vi "Launcher.vi"() -> ()   [LabVIEW 2020]
uses:
  <userlib>/_NEVSTOP/Communicable State Machine(CSM)/_Support/GlobalEvent/GEvt-Convert Filter Rules - v1.0.vi
  <userlib>/_NEVSTOP/Communicable State Machine(CSM)/addons/INI-Static-Variable-Support/_Support/instances/_CSM - Read Log Filter Rules - v1.0.vi
  <userlib>/_NEVSTOP/Communicable State Machine(CSM)/_Support/GlobalEvent/LogFilter/SettingVIs/Set Global CSM Filter.vi
  <userlib>/_NEVSTOP/Communicable State Machine(CSM)/_Support/GlobalEvent/LogFilter/SettingVIs/Set Global LogType Filter.vi
  <userlib>/_NEVSTOP/Communicable State Machine(CSM)/_Support/GlobalEvent/LogFilter/SettingVIs/Set Global State Filter.vi
  <userlib>/_NEVSTOP/Communicable State Machine(CSM)/_Support/GlobalEvent/LogFilter/SettingVIs/Set CSM LogType Filter.vi
  <userlib>/_NEVSTOP/Communicable State Machine(CSM)/_Support/GlobalEvent/LogFilter/SettingVIs/Set CSM State Filter.vi
  <userlib>/_NEVSTOP/Communicable State Machine(CSM)/_Support/GlobalEvent/LogFilter/SettingVIs/Set Global StateType Filter.vi
  <userlib>/_NEVSTOP/Communicable State Machine(CSM)/_Support/GlobalEvent/LogFilter/SettingVIs/Set CSM StateType Filter.vi
  <userlib>/_NEVSTOP/Communicable State Machine(CSM)/addons/INI-Static-Variable-Support/_Support/instances/_CSM - Read File Logger Configuration - v1.0.vi
  src/resource/global-rc-strings.vi
  <userlib>/_NEVSTOP/Communicable State Machine(CSM)/_Support/GlobalEvent/LogFilter/LogFilter.lvclass
  <userlib>/_NEVSTOP/Communicable State Machine(CSM)/addons/Watchdog/CSM Watchdog.lvlib
  <userlib>/_NEVSTOP/Communicable State Machine(CSM)/addons/Logger/CSM File Logger.lvlib
  <userlib>/_NEVSTOP/Communicable State Machine(CSM)/Communicable State Machine.lvlib
  <userlib>/_NEVSTOP/Communicable State Machine(CSM)/addons/INI-Static-Variable-Support/INI-Static-Variable-Support.lvlib
  src/CSMScript-Engine(Lite).lvlib
panel:
  out "Information":string="Load \"csm\"..."
  out "CSMVersion":string="Powered By CSM, Copyright ?2025 NEVSTOP-LAB"
  out "CSMScript(version)":string="CSMScript-Lite"
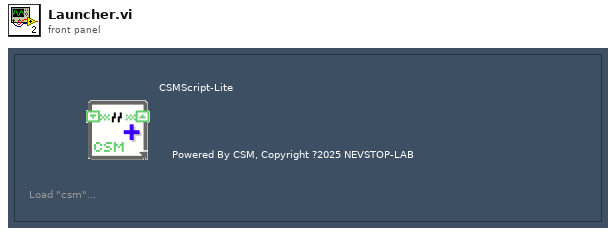
[diagram p1: front panel]
types:
  T1 = cluster{"Enable":bool, "Limit":cluster{"FileSize":i64, "FileNum":i32}, "Timestamp.Format":string, "AutoExit":bool}
  T2 = typedef "Communicable State Machine.lvlib/_CSM_GlobalLog Filter Rules - v1.0.ctl" = cluster{"Global":cluster{"CSM":string[], "LogType":T3[], "State":string[], "StateType":T4[]}, "CSM":cluster{"LogType":cluster{"CSM":string, "LogType":T3}[], "State":cluster{"CSM":string, "State":string}[], "StateType":cluster{"CSM":string, "LogType":T4}[]}}
  T3 = typedef "Communicable State Machine.lvlib/_CSM_GlobalLog_MSG_TYPE.ctl" = enum16{"User Log", "State Change", "Status", "Interrupt", "Register", "Unregister", "Error Log", "Module Created", "Module Destroyed", "Async Message", "No-Rep Async Message", "Sync Message", "AsyncMsg Complete", "SyncMsg Complete"}
  T4 = typedef "Communicable State Machine.lvlib/_CSM_GlobalLog_STATE_TYPE.ctl" = enum16{"State - Internal State", "State - External Message", "State - Response", "State - Complete"}
  T5 = enum32{"Invalid", "Standard", "Closed", "Hidden", "Minimized", "Maximized"}
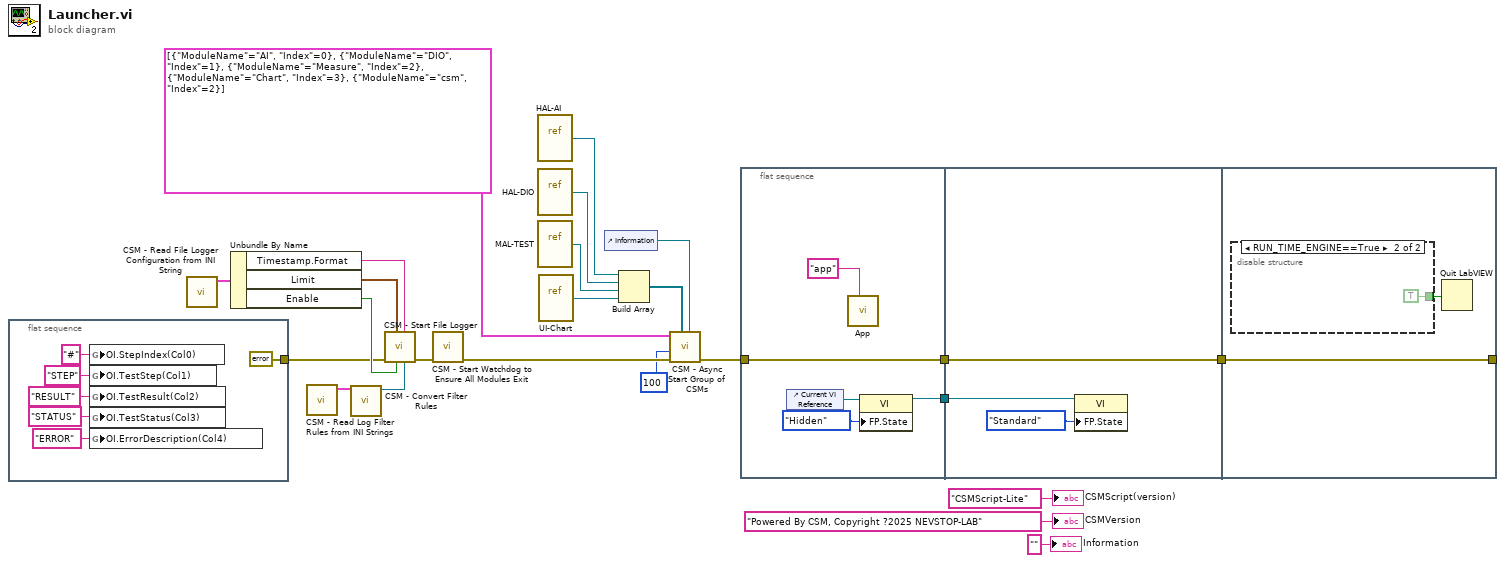
[diagram p0: block diagram]
diagram:
  n1 = flat-sequence {
    tunnel: [errorcluster {"status"=FALSE, "code"=0, "source"=""} ("error in (no error)")] -> w1
    frame #0 {
      n2 = global write "global-rc-strings.vi" "OI.StepIndex(Col0)"("#" ("OI.StepIndex(Col0)")) -> ()
      n3 = global write "global-rc-strings.vi" "OI.TestStep(Col1)"("STEP" ("OI.TestStep(Col1)")) -> ()
      n4 = global write "global-rc-strings.vi" "OI.TestResult(Col2)"("RESULT" ("OI.TestResult(Col2)")) -> ()
      n5 = global write "global-rc-strings.vi" "OI.TestStatus(Col3)"("STATUS" ("OI.TestStatus(Col3)")) -> ()
      n6 = global write "global-rc-strings.vi" "OI.ErrorDescription(Col4)"("ERROR" ("OI.TestStatus(Col3)")) -> ()
    }
  }
  n7 = call-poly <userlib>:"CSM - Read File Logger Configuration from INI String.vi"() -> ("FileLogger Configuration-v1"=w11:T1)  [unwired: 8 in, 1 out]
  n8 = Unbundle By Name(w11) -> ("Timestamp.Format"=w8:string, "Limit"=w9:cluster{"FileSize":i64, "FileNum":i32}, "Enable"=w10:bool)
  n9 = call-poly <userlib>:"CSM - Read Log Filter Rules from INI Strings.vi"() -> ("Rules-v1"=w13:T2)  [unwired: 8 in, 1 out]
  n10 = call-poly <userlib>:"CSM - Convert Filter Rules.vi"("Rules-v1"=w13) -> ("GlobalLogFilter"=w14:refnum<class "LogFilter.lvclass">)  [unwired: 10 in]
  n11 = call <userlib>:"CSM - Start File Logger.vi"("Filter Rules"=w14, "Timestamp Format"=w8, "Enable? (T)"=w10, "Log Limit"=w9, "Error In"=w1) -> ("error out"=w7:errorcluster)  [unwired: 4 in, 2 out]
  n12 = call <userlib>:"CSM - Start Watchdog to Ensure All Modules Exit.vi"("error in (no error)"=w7) -> ("error out"=w21:errorcluster)  [unwired: 10 in]
  n13 = vi-ref "HAL-AI.vi"() -> (w24:refnum<vi>)
  n14 = vi-ref "HAL-DIO.vi"() -> (w23:refnum<vi>)
  n15 = vi-ref "MAL-TEST.vi"() -> (w22:refnum<vi>)
  n16 = vi-ref "UI-Chart.vi"() -> (w15:refnum<vi>)
  n17 = control-ref of="Information"() -> (w3:refnum<vi>)
  n18 = Build Array(w24, w23, w22, w15) -> (w5:refnum<vi>[])
  n19 = call "CSM - Async Start Group of CSMs.vi"("Information"=w3, "Prototypes"=w5, "error in (no error)"=w21, "interval(50ms)"=u32 100, "Module List"=cluster{"ModuleName":string, "Index":i32}[] [{"ModuleName"="AI", "Index"=0}, {"ModuleName"="DIO", "Index"=1}, {"ModuleName"="Measure", "Index"=2}, {"ModuleName"="Chart", "Index"=3}, {"ModuleName"="csm", "Index"=2}]) -> ("error out"=w20:errorcluster)  [unwired: 4 in]
  n20 = flat-sequence {
    tunnel: w20 -> [w35]
    tunnel: [w35] -> w19
    tunnel: [w32] -> w16
    tunnel: w19 -> [w38]
    tunnel: w16 -> [w36]
    tunnel: [w38] -> w12
    tunnel: [w40] -> _
    tunnel: w12 -> [w40]
    frame #0 {
      n21 = control-ref of="Current VI Reference"() -> (w34:refnum<vi>)
      n22 = call "App.vi"("Name(\"\" to use uuid)"="app" ("Name(\"\" to use uuid)")) -> ()  [unwired: 11 in]
      n23 = property class="VI"(reference=w34, "FP.State"=T5."Hidden" ("Front Panel Window:State")) -> (reference out=w32:refnum<vi>)  [unwired: 1 in, 1 out]
    }
    frame #1 {
      n24 = property class="VI"(reference=w36, "FP.State"=T5."Standard" ("Front Panel Window:State")) -> ()  [unwired: 1 in, 2 out]
    }
    frame #2 {
      n25 = disable-structure shown="RUN_TIME_ENGINE==True" {
        disable-tunnel: [_ TRUE ("quit? (T)")] -> w39
        frame condition #0 (active) {
        }
        frame condition #1 {
        }
      }
      n26 = Quit LabVIEW(quit? (T)=w39) -> ()
    }
  }
  "CSMScript(version)" <- "CSMScript-Lite" ("String to Prepend to Source (\"\")")
  "CSMVersion" <- "Powered By CSM, Copyright ?2025 NEVSTOP-LAB" ("String to Prepend to Source (\"\")")
  "Information" <- "" ("Information")
